vi "Raw.vi"(8 "error in (no error)":errorcluster, 10 "Map":i32[](array[numeric]), 11 "Raw In":refnum<class "Cross.lvclass">) -> (0 "error out":errorcluster, 1 "Direction":T1, 2 "Action":T2, 3 "Raw Out":refnum<class "Cross.lvclass">, 4 "Replicated Class":refnum<class "Cross.lvclass">)   [LabVIEW 2015, in "Cross.lvclass"]
uses:
  Cross.lvclass
  Type Defs/Action Enum.ctl
  Type Defs/Direction Enum.ctl
  Type Defs/SB Type Defs.lvlib
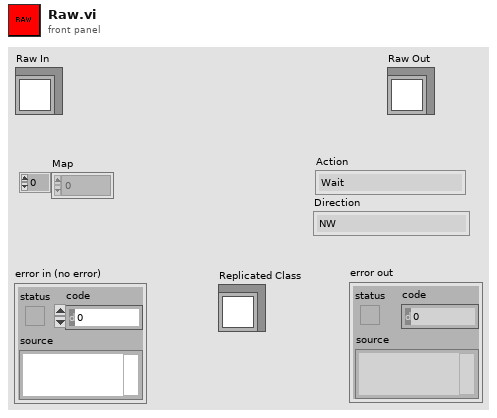
[diagram p1: front panel]
types:
  T1 = typedef "SB Type Defs.lvlib/Direction Enum.ctl" = enum16{"NW", "N", "NE", "E", "SE", "S", "SW", "W"}
  T2 = typedef "SB Type Defs.lvlib/Action Enum.ctl" = enum16{"Wait", "Move", "Attack", "Replicate"}
  T3 = enum16{"Raw", "Spawner", "Builder", "Gunner", "Fighter"}
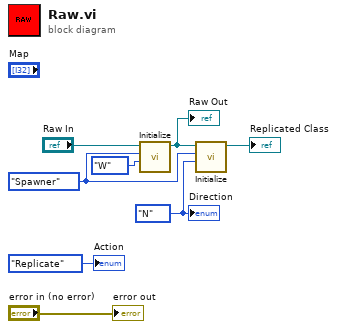
[diagram p0: block diagram]
diagram:
  w4 = Direction_Enum."N" ("Direction")
  w5 = T3."Spawner" ("Job")
  n1 = call "Initialize.vi"("Direction"=Direction_Enum."W", "Job"=w5, "Runner in"="Raw In") -> ("Runner out"=w2:refnum<class "Cross.lvclass">)  [unwired: 8 in]
  "Raw Out" <- w2
  n2 = call "Initialize.vi"("Direction"=w4, "Job"=w5, "Runner in"=w2) -> ("Runner out"=→"Replicated Class":refnum<class "Cross.lvclass">)  [unwired: 8 in]
  "error out" <- "error in (no error)"
  "Action" <- Action_Enum."Replicate" ("Action")
  "Direction" <- w4
